vi "VibSystem1Signals.vi"(8 "sampling info":cluster{"Fs":dbl, "#s":dbl}={"Fs"=10000.0, "#s"=10000.0} {"Fs" format="%.2p"}, 9 "Temperature Channel Voltage In":dbl, 10 "Frequency":dbl, 11 "Constant Amplitudes?":bool) -> (1 "Temperature Channel Voltage Out":dbl, 3 "Signals":waveform(dbl)[](array[waveform]))   [LabVIEW 2017]
uses:
  <vilib>/measure/NI_MABase.lvlib
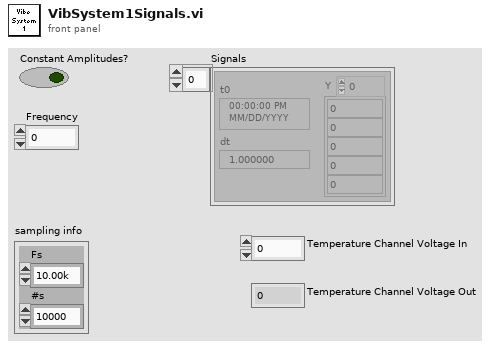
[diagram p1: front panel]
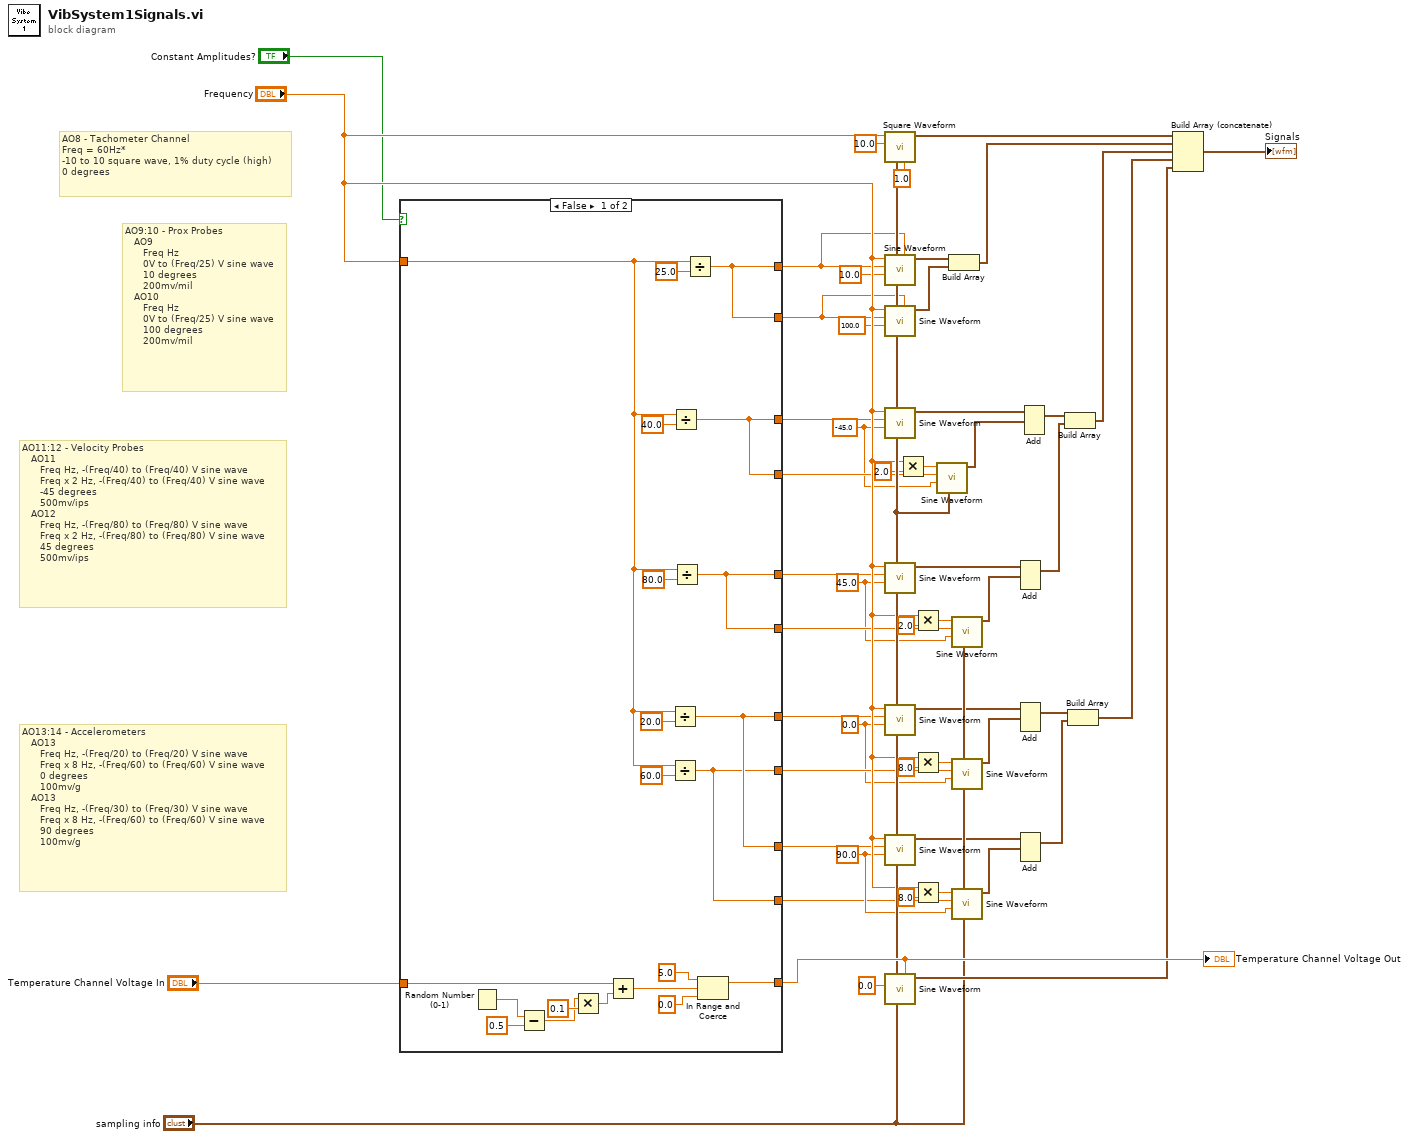
[diagram p0: block diagram]
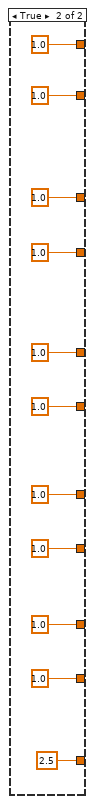
[diagram p2: hidden frame]
diagram:
  w42 = 90.0 ("phase")
  w33 = 0.0 ("phase")
  w15 = 45.0 ("phase")
  w14 = -45.0 ("phase")
  # "AO13:14 - Accelerometers\n   AO13\n      Freq Hz, -(Freq/20) to (Freq/20) V sine wave\n      Freq x 8 Hz, -(Freq/60) to (Freq/60) V sine wave\n      0 degrees\n      100mv/g\n   AO13\n      Freq Hz, -(Freq/30) to (Freq/30) V sine wave\n      Freq x 8 Hz, -(Freq/60) to (Freq/60) V sine wave\n      90 degrees\n      100mv/g"
  # "AO11:12 - Velocity Probes\n   AO11\n      Freq Hz, -(Freq/40) to (Freq/40) V sine wave\n      Freq x 2 Hz, -(Freq/40) to (Freq/40) V sine wave\n      -45 degrees\n      500mv/ips\n   AO12\n      Freq Hz, -(Freq/80) to (Freq/80) V sine wave\n      Freq x 2 Hz, -(Freq/80) to (Freq/80) V sine wave\n      45 degrees\n      500mv/ips"
  # "AO9:10 - Prox Probes\n   AO9\n      Freq Hz\n      0V to (Freq/25) V sine wave\n      10 degrees\n      200mv/mil\n   AO10\n      Freq Hz\n      0V to (Freq/25) V sine wave\n      100 degrees\n      200mv/mil"
  # "AO8 - Tachometer Channel\nFreq = 60Hz*\n-10 to 10 square wave, 1% duty cycle (high)\n0 degrees"
  n1 = case shown="False" "Constant Amplitudes?" {
    tunnel: [w72 1.0] -> w23
    tunnel: [w72 1.0] -> w24
    tunnel: [w69 1.0] -> w21
    tunnel: [w69 1.0] -> w22
    tunnel: [w68 1.0] -> w25
    tunnel: [w68 1.0] -> w26
    tunnel: "Frequency" -> [w65 _]
    tunnel: [w64 1.0] -> w36
    tunnel: [w63 1.0] -> w37
    tunnel: [w64 1.0] -> w39
    tunnel: [w63 1.0] -> w38
    tunnel: "Temperature Channel Voltage In" -> [w54 _]
    tunnel: [w60 2.5 ("upper limit")] -> w52
    frame False {
      n2 = Random Number (0-1)() -> (number: 0 to 1=w58:dbl)
      n3 = Subtract(x=w58, y=0.5) -> (x-y=w56:dbl)
      n4 = Multiply(x=w56, y=0.1) -> (x*y=w55:dbl)
      n5 = Add(x=w54, y=w55) -> (x+y=w53:dbl)
      n6 = Divide(x=w65, y=20.0) -> (x/y=w64:dbl)
      n7 = Divide(x=w65, y=60.0) -> (x/y=w63:dbl)
      n8 = Divide(x=w65, y=40.0) -> (x/y=w69:dbl)
      n9 = Divide(x=w65, y=80.0) -> (x/y=w68:dbl)
      n10 = Divide(x=w65, y=25.0) -> (x/y=w72:dbl)
      n11 = In Range and Coerce(upper limit=5.0, x=w53, lower limit=0.0) -> (coerced(x)=w60:dbl)  [unwired: 1 out]
    }
    frame True {
    }
  }
  "Temperature Channel Voltage Out" <- w52
  n12 = call <vilib>:"Square Waveform.vi"("duty cycle (%)"=1.0, "sampling info"="sampling info", "amplitude"=10.0, "frequency"="Frequency") -> ("signal out"=w6:waveform(dbl))  [unwired: 6 in, 1 out]
  n13 = call <vilib>:"Sine Waveform.vi"("offset"=w23, "sampling info"="sampling info", "phase"=10.0, "amplitude"=w23, "frequency"="Frequency") -> ("signal out"=w19:waveform(dbl))  [unwired: 5 in, 1 out]
  n14 = call <vilib>:"Sine Waveform.vi"("offset"=w24, "sampling info"="sampling info", "phase"=100.0, "amplitude"=w24, "frequency"="Frequency") -> ("signal out"=w20:waveform(dbl))  [unwired: 5 in, 1 out]
  n15 = call <vilib>:"Sine Waveform.vi"("sampling info"="sampling info", "phase"=w14, "amplitude"=w21, "frequency"="Frequency") -> ("signal out"=w11:waveform(dbl))  [unwired: 6 in, 1 out]
  n16 = call <vilib>:"Sine Waveform.vi"("sampling info"="sampling info", "phase"=w15, "amplitude"=w25, "frequency"="Frequency") -> ("signal out"=w17:waveform(dbl))  [unwired: 6 in, 1 out]
  n17 = call <vilib>:"Sine Waveform.vi"("sampling info"="sampling info", "phase"=w33, "amplitude"=w36, "frequency"="Frequency") -> ("signal out"=w31:waveform(dbl))  [unwired: 6 in, 1 out]
  n18 = call <vilib>:"Sine Waveform.vi"("sampling info"="sampling info", "phase"=w42, "amplitude"=w39, "frequency"="Frequency") -> ("signal out"=w44:waveform(dbl))  [unwired: 6 in, 1 out]
  n19 = call <vilib>:"Sine Waveform.vi"("offset"=w52, "sampling info"="sampling info", "amplitude"=0.0) -> ("signal out"=w51:waveform(dbl))  [unwired: 7 in, 1 out]
  n20 = Multiply(x="Frequency", y=2.0) -> (x*y=w8:dbl)
  n21 = Multiply(x="Frequency", y=2.0) -> (x*y=w13:dbl)
  n22 = Multiply(x="Frequency", y=8.0) -> (x*y=w34:dbl)
  n23 = Multiply(x="Frequency", y=8.0) -> (x*y=w41:dbl)
  n24 = call <vilib>:"Sine Waveform.vi"("sampling info"="sampling info", "phase"=w14, "amplitude"=w22, "frequency"=w8) -> ("signal out"=w10:waveform(dbl))  [unwired: 6 in, 1 out]
  n25 = Build Array(w19, w20) -> (w29:waveform(dbl)[])
  n26 = call <vilib>:"Sine Waveform.vi"("sampling info"="sampling info", "phase"=w15, "amplitude"=w26, "frequency"=w13) -> ("signal out"=w16:waveform(dbl))  [unwired: 6 in, 1 out]
  n27 = call <vilib>:"Sine Waveform.vi"("sampling info"="sampling info", "phase"=w33, "amplitude"=w37, "frequency"=w34) -> ("signal out"=w32:waveform(dbl))  [unwired: 6 in, 1 out]
  n28 = call <vilib>:"Sine Waveform.vi"("sampling info"="sampling info", "phase"=w42, "amplitude"=w38, "frequency"=w41) -> ("signal out"=w43:waveform(dbl))  [unwired: 6 in, 1 out]
  n29 = Add(1:w16, 2:w17) -> (0:w28:waveform(dbl))  [unwired: 1 in, 1 out]
  n30 = Add(1:w32, 2:w31) -> (0:w46:waveform(dbl))  [unwired: 1 in, 1 out]
  n31 = Add(1:w43, 2:w44) -> (0:w47:waveform(dbl))  [unwired: 1 in, 1 out]
  n32 = Add(1:w10, 2:w11) -> (0:w27:waveform(dbl))  [unwired: 1 in, 1 out]
  n33 = Build Array(w27, w28) -> (w30:waveform(dbl)[])
  n34 = Build Array(w46, w47) -> (w48:waveform(dbl)[])
  n35 = Build Array (concatenate)(w6, w29, w30, w48, w51) -> (→"Signals":waveform(dbl)[])
